vi "From Serial Form.vi"(6 "Serial Version":T1, 10 "Deserializer in":refnum<class "Deserializer.lvclass">, 11 "Alicat Controller in":refnum<class "Alicat Controller.lvclass">) -> (0 "error out":errorcluster, 2 "Deserializer out":refnum<class "Deserializer.lvclass">, 3 "Alicat Controller out":refnum<class "Alicat Controller.lvclass">)   [LabVIEW 2012, in "Alicat.lvlib" / "Alicat Controller.lvclass"]
uses:
  Alicat Controller.lvclass
  <userlib>/Serialization/Deserializer/Deserializer.lvclass
  <userlib>/Serialization/Serialization Common/Serial Version.ctl
  Alicat.lvclass
  Alicat Controller.lvclass/Alicat Controller.ctl
  <userlib>/Serialization/Serializable/Remove Double.vi
  <userlib>/Serialization/Serializable/Serializable.lvclass
  <userlib>/Serialization/Serialization Common/Serialization Common.lvlib
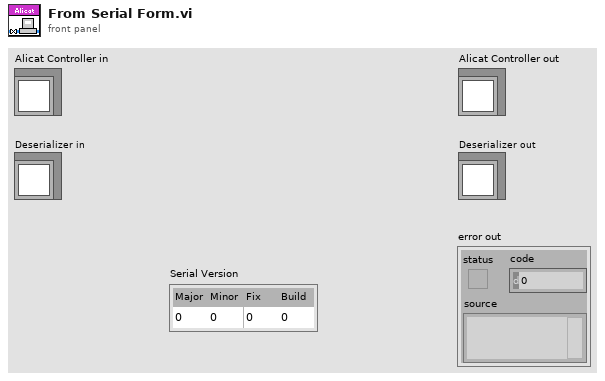
[diagram p1: front panel]
types:
  T1 = typedef "Serialization Common.lvlib/Serial Version.ctl" = cluster{"Major":u16, "Minor":u16, "Fix":u16, "Build":u16}
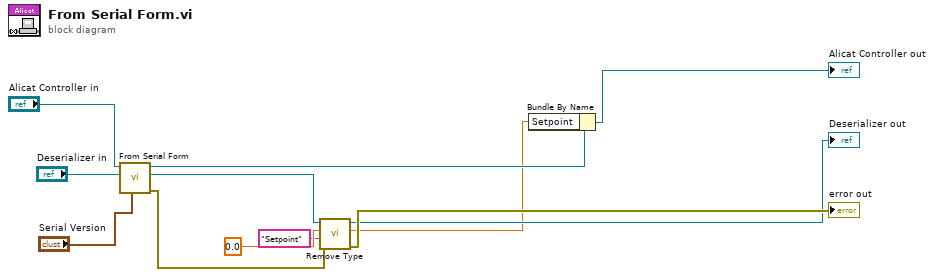
[diagram p0: block diagram]
diagram:
  n1 = call-parent "From Serial Form.vi"("Serial Version"="Serial Version", "Deserializer in"="Deserializer in", "Alicat in"="Alicat Controller in") -> ("error out"=w5:errorcluster, "Deserializer out"=w7:refnum<class "Deserializer.lvclass">, "Alicat out"=w9:refnum<class "Alicat Controller.lvclass">)  [unwired: 6 in]
  n2 = call-poly <userlib>:"Remove Type.vi"("error in (no error)"=w5, "Name"="Setpoint", "Default Value"=0.0, "Deserializer in"=w7) -> ("error out"=→"error out":errorcluster, "Numeric"=w1:dbl, "Deserializer out"=→"Deserializer out":refnum<class "Deserializer.lvclass">)  [unwired: 4 in, 1 out]
  n3 = Bundle By Name(cluster=w9, "Setpoint"=w1) -> (→"Alicat Controller out":refnum<class "Alicat Controller.lvclass">)
